vi "TestCase.vi"(1 "name":string) -> (0 "TestCase out":refnum<class "TestCase.lvclass">)   [LabVIEW 2014, in "TestCase.lvclass"]
uses:
  TestCase.lvclass
  TestCase.lvclass/TestCase.ctl
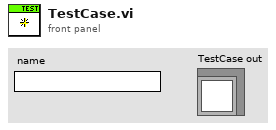
[diagram p1: front panel]
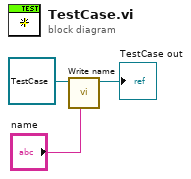
[diagram p0: block diagram]
diagram:
  n1 = call "Write name.vi"("name"="name", "TestCase in"=refnum<class "TestCase.lvclass"> refnum) -> ("TestCase out"=→"TestCase out":refnum<class "TestCase.lvclass">)  [unwired: 7 in]
